vi "SAOMM-Cursor2ROI.vi"(1 "ImgRef":refnum<vi>, 5 "CursorX":dbl, 9 "CursorY":dbl, 12 "ROIWidth":u16, 13 "ROIHeight":u16) -> (4 "XÉtoile":dbl, 6 "YÉtoile":dbl, 10 "ROIXOffset":u16, 15 "ROIYOffset":u16)   [LabVIEW 2011]
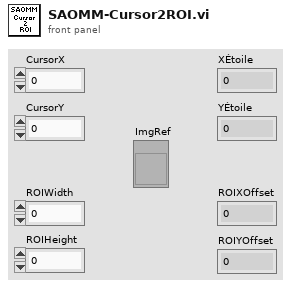
[diagram p1: front panel]
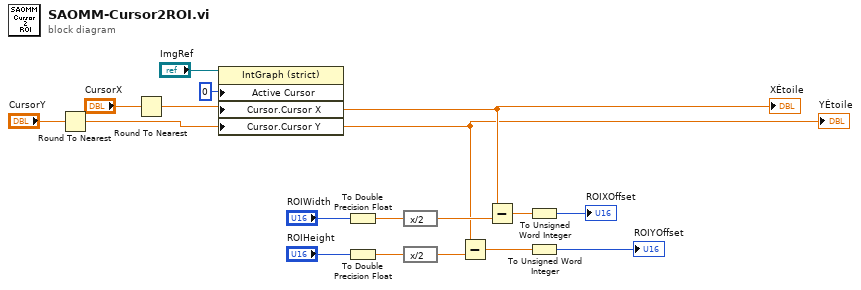
[diagram p0: block diagram]
diagram:
  n1 = Round To Nearest(number="CursorY") -> (nearest integer value=w3:dbl)
  "YÉtoile" <- w3
  n2 = Round To Nearest(number="CursorX") -> (nearest integer value=w4:dbl)
  "XÉtoile" <- w4
  n3 = property class="IntGraph (strict)"(reference="ImgRef", "Active Cursor"=u32 0, "Cursor.Cursor X"=w4, "Cursor.Cursor Y"=w3) -> ()  [unwired: 1 in, 2 out]
  n4 = To Double Precision Float(number="ROIWidth") -> (double precision float=w7:dbl)
  n5 = To Double Precision Float(number="ROIHeight") -> (double precision float=w8:dbl)
  n6 = expression code="x/2"(w7) -> (w9:dbl)
  n7 = expression code="x/2"(w8) -> (w10:dbl)
  n8 = Subtract(x=w3, y=w10) -> (x-y=w12:dbl)
  n9 = Subtract(x=w4, y=w9) -> (x-y=w11:dbl)
  n10 = To Unsigned Word Integer(number=w11) -> (unsigned 16bit integer=→"ROIXOffset":u16)
  n11 = To Unsigned Word Integer(number=w12) -> (unsigned 16bit integer=→"ROIYOffset":u16)
